vi "generador_de_datos.vi"() -> ()   [LabVIEW 2019]
panel:
  in  "Ring":u16(ring) items=["Triangular", "Cuadrada", "Diente de Sierra", "Seno"]
  out "Array 2":string[](array[string])
  in  "Ubicación del archivo":path
  out "Array":string[](array[string])
  out "Boolean array":bool[](array[boolean])
  in  "stop":bool
  out "Ploter":dbl(graph)
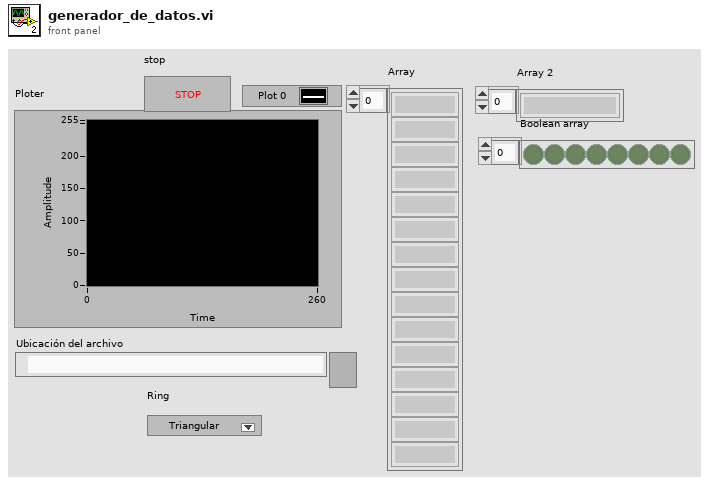
[diagram p1: front panel]
types:
  T1 = enum16{"open", "replace", "create", "open or create", "replace or create", "replace or create with confirmation"}
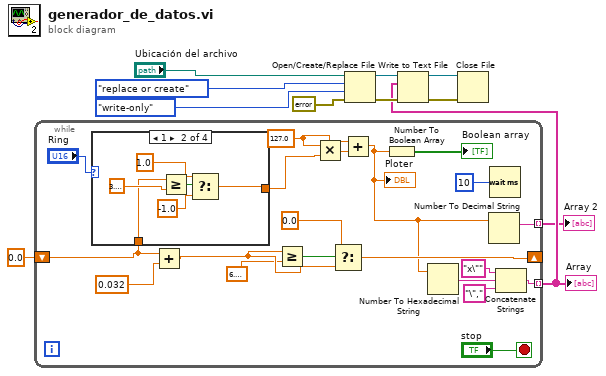
[diagram p0: block diagram]
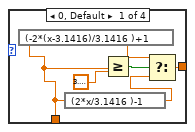
[diagram p2: hidden frame]
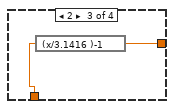
[diagram p3: hidden frame]
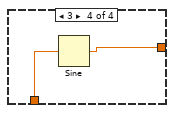
[diagram p4: hidden frame]
diagram:
  n1 = while {
    shift-right: [w26] -> _
    shift-left: 0.0 -> [w13]
    tunnel: [w19] -> w2 mode=indexing
    tunnel: [w17] -> w1 mode=indexing
    stop <- "stop" stop-if-true
    w22 = 127.0 ("x")
    n2 = case shown="1" "Ring" {
      tunnel: [w34 w38 w45 w47] -> w14
      tunnel: w13 -> [w33 w39 w44 w46]
      frame 0, Default {
        n3 = expression code="(-2*(x-3.1416)/3.1416 )+1"(w33) -> (w37:dbl)
        n4 = expression code="(2*x/3.1416 )-1"(w33) -> (w32:dbl)
        n5 = Greater Or Equal?(x=w33, y=3.141592653589793) -> (x >= y?=w36:bool)
        n6 = Select(t=w37, s=w36, f=w32) -> (s? t:f=w34:dbl)
      }
      frame 1 {
        n7 = Greater Or Equal?(x=w39, y=3.141592653589793) -> (x >= y?=w43:bool)
        n8 = Select(t=1.0, s=w43, f=-1.0) -> (s? t:f=w38:dbl)
      }
      frame 2 {
        n9 = expression code="(x/3.1416 )-1"(w44) -> (w45:dbl)
      }
      frame 3 {
        n10 = Sine(x=w46) -> (sin(x)=w47:dbl)
      }
    }
    n11 = Add(x=w13, y=0.032) -> (x+y=w27:dbl)
    n12 = Greater Or Equal?(x=w27, y=6.283185307179586) -> (x >= y?=w30:bool)
    n13 = Multiply(x=w22, y=w14) -> (x*y=w24:dbl)
    n14 = Select(t=0.0, s=w30, f=w27) -> (s? t:f=w26:dbl)
    n15 = Add(x=w22, y=w24) -> (x+y=w15:dbl)
    "Ploter" <- w15
    n16 = Number To Boolean Array(number=w15) -> (Boolean array=→"Boolean array":bool[])
    n17 = Number To Hexadecimal String(2:w15) -> (0:w20:string)  [unwired: 1 in]
    n18 = Number To Decimal String(number=w15) -> (decimal integer string=w17:string)  [unwired: 1 in]
    n19 = Wait (ms)(milliseconds to wait=u32 10) -> ()  [unwired: 1 out]
    n20 = Concatenate Strings("x\"", w20, "\",") -> (w19:string)
  }
  "Array" <- w2
  "Array 2" <- w1
  n21 = Open/Create/Replace File(file path (use dialog)="Ubicación del archivo", error in=errorcluster {"status"=FALSE, "code"=0, "source"=""}, operation (0:open)=T1."replace or create", access (0:read/write)=enum16{"read/write", "read-only", "write-only"}."write-only") -> (refnum out=w5:refnum<file>, error out=w6:errorcluster)  [unwired: 2 in, 1 out]
  n22 = Write to Text File(file (use dialog)=w5, text=w2, error in=w6) -> (refnum out=w3:refnum<file>, error out=w4:errorcluster)  [unwired: 1 in, 1 out]
  n23 = Close File(refnum=w3, error in=w4) -> ()  [unwired: 2 out]
